vi "PR_Update_Assemble_time .vi"(8 "error in (no error)":errorcluster, 10 "barcode":string="984132195", 11 "DBlink":string="Driver={ODBC Driver 17 for SQL Server};Server=localhost\\SQLEXPRESS;Database=ZDX201;UID=labview;PWD=Dsa@54137926") -> (0 "error out":errorcluster, 2 "前一製程結果":string, 3 "給PLC":i32)   [LabVIEW 2019]
uses:
  <vilib>/addons/database/Connection.llb/DB Tools Open Connec (String).vi
  <vilib>/addons/database/_DB Variant To Data/Database Variant To Data.xnode
  <vilib>/addons/database/NI_Database_API.lvlib
panel:
  out "result":string
  out "data":cluster{string}[](array[cluster])
  out "concatenated string":string="WHERE [barcode]='984132195' and [pos]='B'"
  in  "columns":string[](array[string])=["assemble_time", "update_time"]
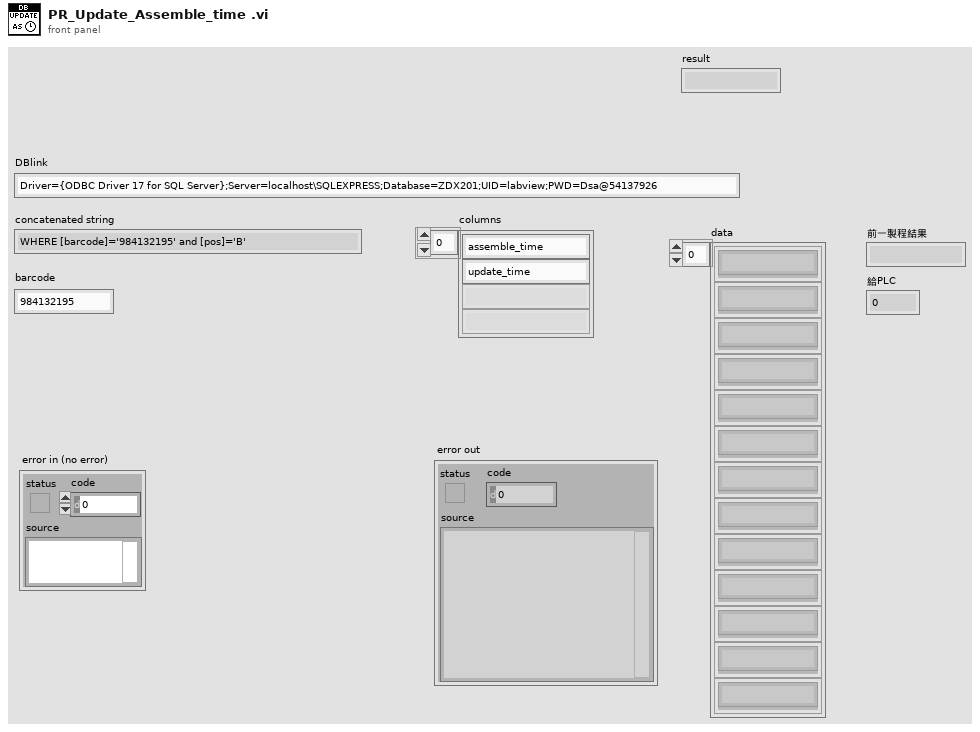
[diagram p1: front panel]
types:
  T1 = cluster{"assemble_time":timestamp, "update_time":timestamp}
  T2 = typedef "NI_Database_API.lvlib/Conn ObjectReference.ctl" = refnum<k1>
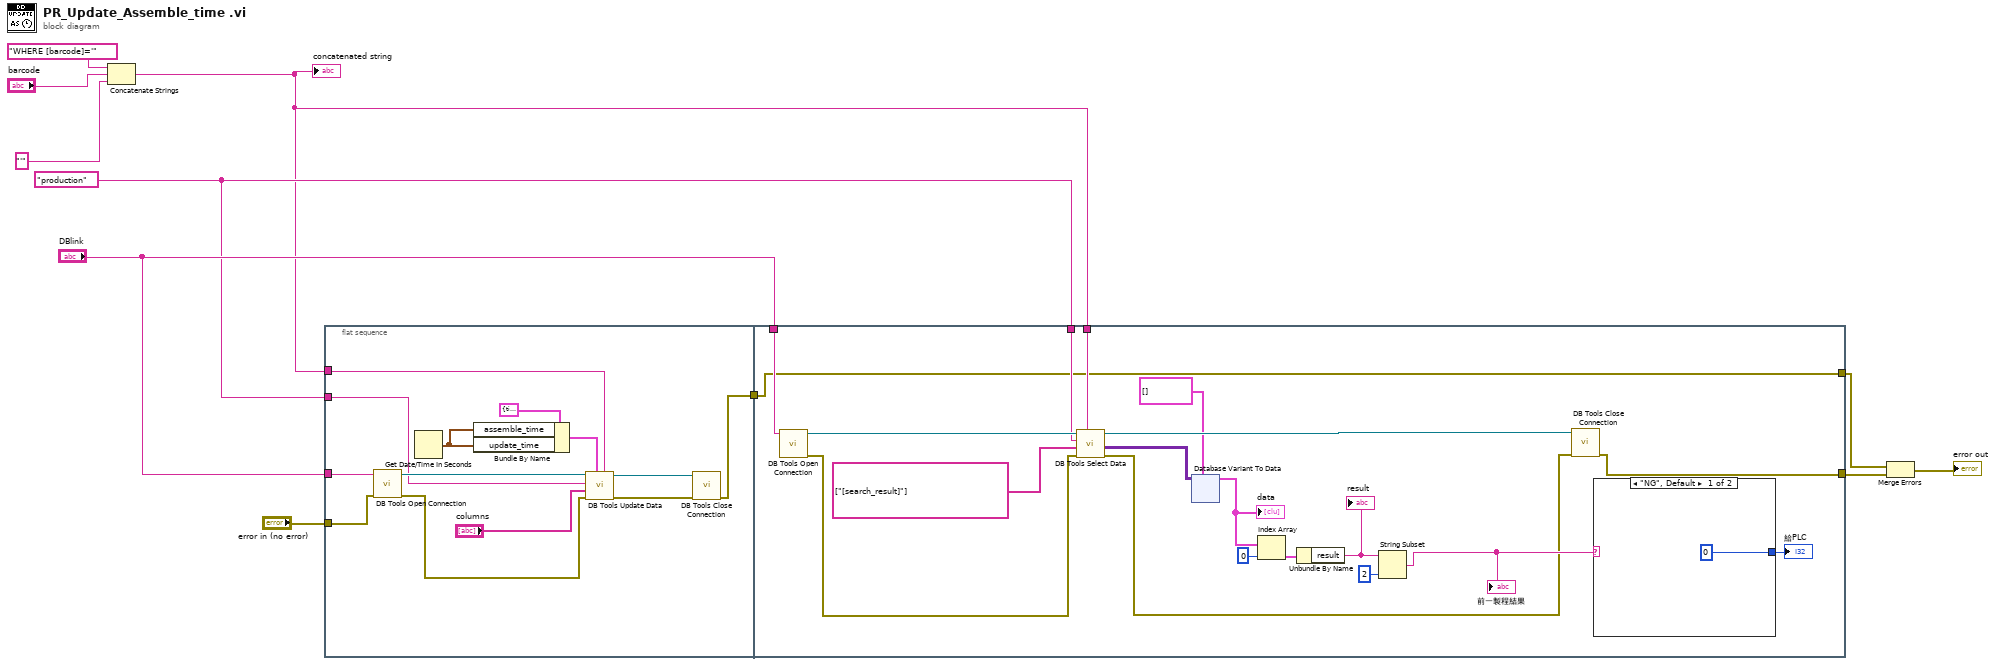
[diagram p0: block diagram]
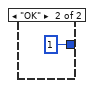
[diagram p2: hidden frame]
diagram:
  w6 = "production" ("table")
  n1 = Concatenate Strings("WHERE [barcode]='", "barcode", "'" ("string")) -> (w5:string)
  "concatenated string" <- w5
  n2 = flat-sequence {
    tunnel: "error in (no error)" -> [w24]
    tunnel: "DBlink" -> [w15]
    tunnel: w6 -> [w14]
    tunnel: w5 -> [w13]
    tunnel: [w12] -> w2
    tunnel: "DBlink" -> [w29]
    tunnel: w6 -> [w28]
    tunnel: w5 -> [w27]
    tunnel: [w26] -> w3
    tunnel: w2 -> [w25]
    tunnel: [w25] -> w1
    frame #0 {
      n3 = call-poly <vilib>:"DB Tools Open Connection.vi"("error in (no error)"=w24, "connection information"=w15) -> ("error out"=w22:errorcluster, "connection reference"=w20:T2)  [unwired: 6 in]
      n4 = Get Date/Time In Seconds() -> (seconds since 1Jan1904=w17:timestamp)
      n5 = Bundle By Name(cluster=T1 {"assemble_time"=timestamp(0 s since 1904-01-01), "update_time"=timestamp(0 s since 1904-01-01)}, "assemble_time"=w17, "update_time"=w17) -> (w16:T1)
      n6 = call <vilib>:"DB Tools Update Data.vi"("condition"=w13, "data"=w16, "error in (no error)"=w22, "columns"="columns", "table"=w14, "connection reference"=w20) -> ("error out"=w23:errorcluster, "connection reference out"=w21:T2)  [unwired: 4 in]
      n7 = call <vilib>:"DB Tools Close Connection.vi"("error in (no error)"=w23, "connection reference"=w21) -> ("error out"=w12:errorcluster)  [unwired: 5 in]
    }
    frame #1 {
      n8 = call-poly <vilib>:"DB Tools Open Connection.vi"("connection information"=w29) -> ("error out"=w35:errorcluster, "connection reference"=w34:T2)  [unwired: 7 in]
      n9 = call <vilib>:"DB Tools Select Data.vi"("condition"=w27, "error in (no error)"=w35, "columns"=string[] ["[search_result]"] ("columns 2"), "table"=w28, "connection reference"=w34) -> ("error out"=w37:errorcluster, "data"=w38:variant[][], "connection reference out"=w36:T2)  [unwired: 1 in]
      n10 = xnode "Database Variant To Data"("database variant"=w38, "type"=cluster{"result":string}[] [] ("Region number")) -> ("data"=w39:cluster{"result":string}[])  [unwired: 1 in, 1 out]
      "data" <- w39
      n11 = Index Array(array=w39, index=0) -> (element=w40:cluster{"result":string})
      n12 = Unbundle By Name(w40) -> ("result"=w42:string)
      "result" <- w42
      n13 = String Subset(string=w42, length (rest)=2 ("length (rest)")) -> (substring=w43:string)  [unwired: 1 in]
      "前一製程結果" <- w43
      n14 = call <vilib>:"DB Tools Close Connection.vi"("error in (no error)"=w37, "connection reference"=w36) -> ("error out"=w26:errorcluster)  [unwired: 5 in]
      n15 = case shown="\"NG\", Default" w43 {
        tunnel: [0 1] -> w41
        frame "NG", Default {
        }
        frame "OK" {
        }
      }
      "給PLC" <- w41
    }
  }
  n16 = Merge Errors(w1, w3) -> (→"error out":errorcluster)
